vi "GetBoard.vi"(8 "error in (no error)":errorcluster, 11 "object in":refnum<class "Board.lvclass">) -> (0 "error out":errorcluster, 1 "BoardDrawing":picture[][](array[picture]), 2 "position":string, 3 "object out":refnum<class "Board.lvclass">)   [LabVIEW 2020, in "Board.lvclass"]
uses:
  Board.lvclass
  Board.lvclass/Board.ctl
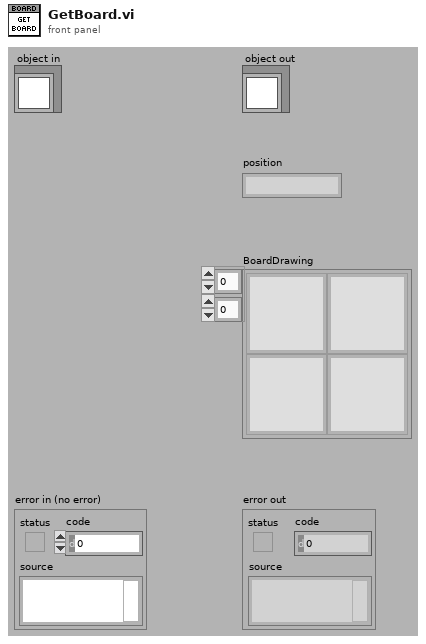
[diagram p1: front panel]
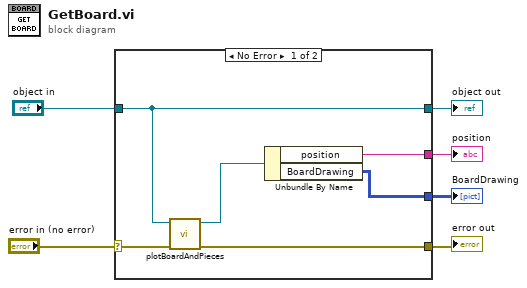
[diagram p0: block diagram]
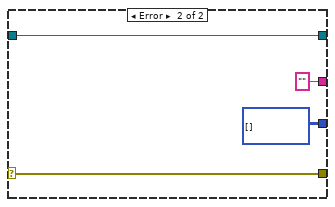
[diagram p2: hidden frame]
diagram:
  n1 = case shown="No Error" "error in (no error)" {
    selector: "error in (no error)" -> [w8 w16]
    tunnel: [w7 w16] -> w5
    tunnel: [w10 w15] -> w3
    tunnel: "object in" -> [w10 w15]
    tunnel: [w12 "" ("board")] -> w2
    tunnel: [w11 picture[][] [] ("BoardDrawing")] -> w1
    frame No Error {
      n2 = call-dynamic "plotBoardAndPieces.vi"("error in (no error)"=w8, "object in"=w10) -> ("error out"=w7:errorcluster, "object out"=w9:refnum<class "Board.lvclass">)  [unwired: 8 in]
      n3 = Unbundle By Name(w9) -> ("position"=w12:string, "BoardDrawing"=w11:picture[][])
    }
    frame Error {
    }
  }
  "error out" <- w5
  "object out" <- w3
  "position" <- w2
  "BoardDrawing" <- w1
